vi "WebCAM_Init.vi"(8 "error in (no error)":errorcluster, 10 "PictureBox 2":refnum<k24>(container) caption="PictureBox ------", 11 "Window Title":string="Title") -> (0 "error out":errorcluster, 2 "error initialising":bool, 3 "hwnd":u32, 4 "picture boxx Handle":refnum<k24>)   [LabVIEW 2011]
uses:
  System.Windows.Forms
  user32.dll
  avicap32.dll
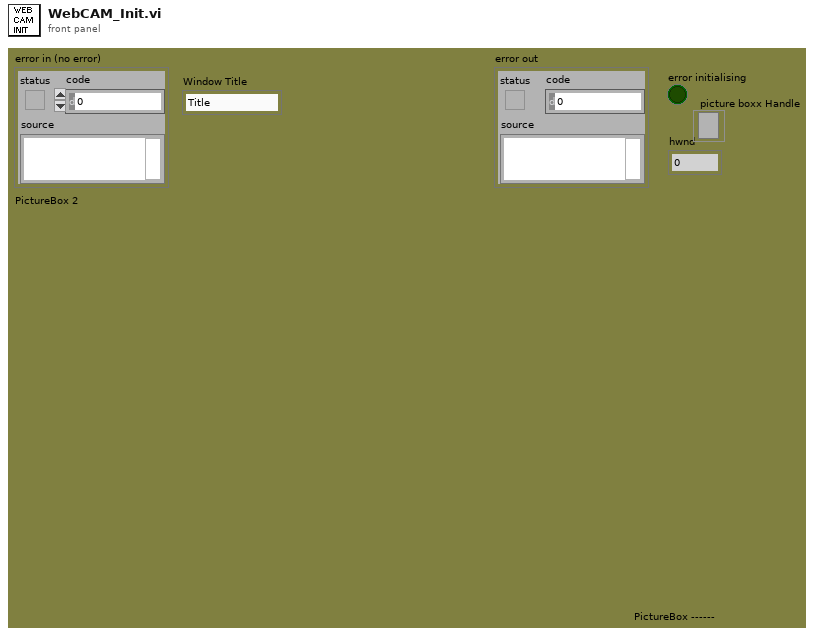
[diagram p1: front panel]
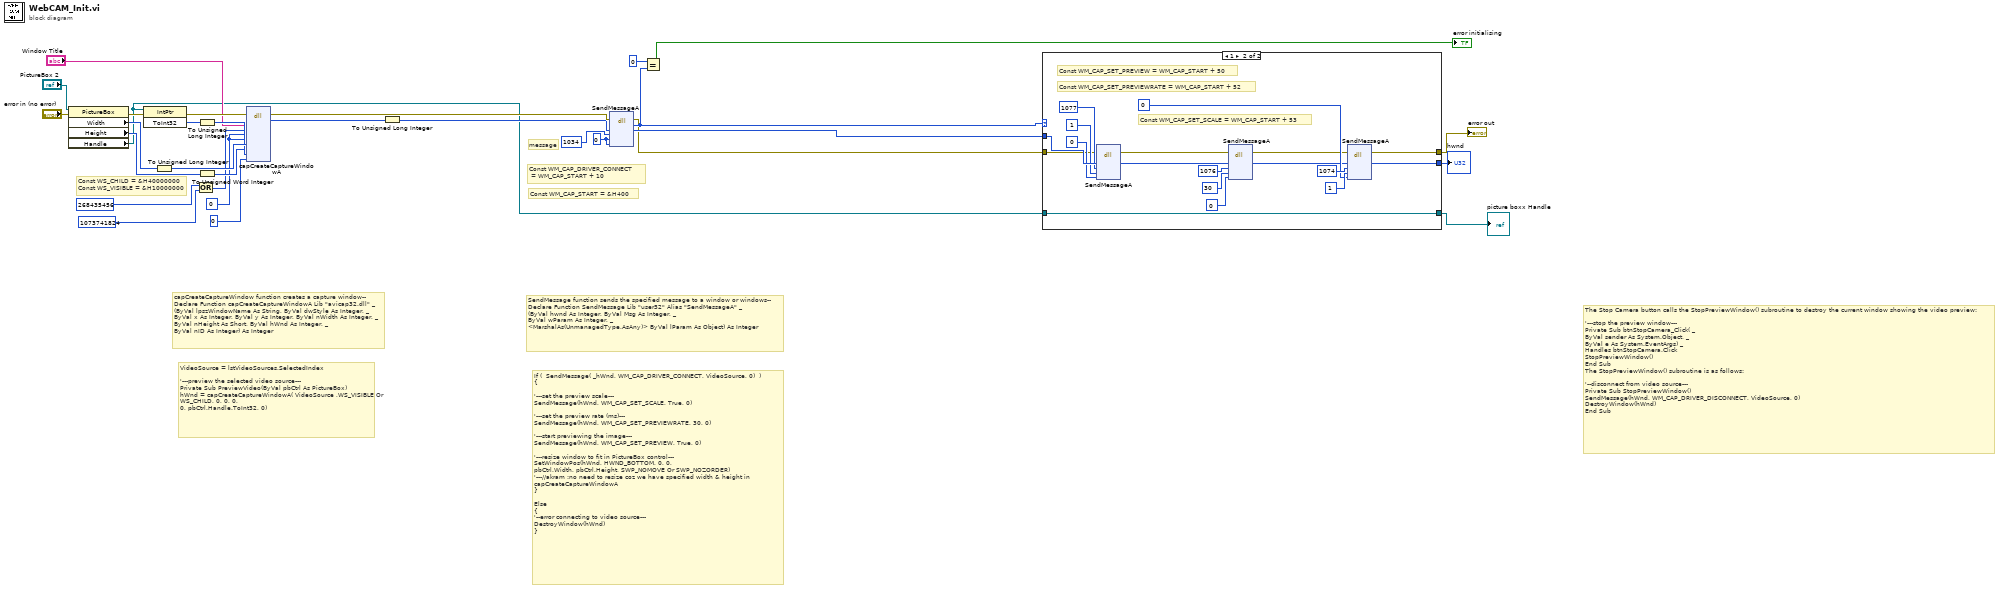
[diagram p0: block diagram]
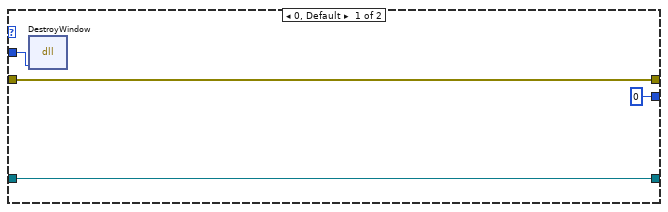
[diagram p2: hidden frame]
diagram:
  w15 = u32 0 ("wParam")
  w18 = u32 0 ("y")
  # "The Stop Camera button calls the StopPreviewWindow() subroutine to destroy the current window showing the video preview:\n\n'---stop the preview window---\nPrivate Sub btnStopCamera_Click( _\nByVal sender As System.Object, _\nByVal e As System.EventArgs) _\nHandles btnStopCamera.Click\nStopPreviewWindow()\nEnd Sub\nThe StopPreviewWindow() subroutine is as follows:\n\n'--disconnect from video source---\nPrivate Sub StopPreviewWindow()\nSendMessage(hWnd, WM_CAP_DRIVER_DISCONNECT, VideoSource, 0)\nDestroyWindow(hWnd)\nEnd Sub"
  # "If (  SendMessage( _hWnd, WM_CAP_DRIVER_CONNECT, VideoSource, 0)  )\n{\n\n'---set the preview scale---\nSendMessage(hWnd, WM_CAP_SET_SCALE, True, 0)\n\n'---set the preview rate (ms)---\nSendMessage(hWnd, WM_CAP_SET_PREVIEWRATE, 30, 0)\n\n'---start previewing the image---\nSendMessage(hWnd, WM_CAP_SET_PREVIEW, True, 0)\n\n'---resize window to fit in PictureBox control---\nSetWindowPos(hWnd, HWND_BOTTOM, 0, 0, \npbCtrl.Width, pbCtrl.Height, SWP_NOMOVE Or SWP_NOZORDER)\n'---//akram :no need to resize coz we have specified width & height in capCreateCaptureWindowA\n}\n\nElse\n{\n'--error connecting to video source---\nDestroyWindow(hWnd)\n}"
  # "Const WM_CAP_START = &H400"
  # "Const WM_CAP_DRIVER_CONNECT\n = WM_CAP_START + 10"
  # "VideoSource = lstVideoSources.SelectedIndex\n\n'---preview the selected video source---\nPrivate Sub PreviewVideo(ByVal pbCtrl As PictureBox)\nhWnd = capCreateCaptureWindowA( VideoSource ,WS_VISIBLE Or WS_CHILD, 0, 0, 0, \n0, pbCtrl.Handle.ToInt32, 0)"
  # "message"
  # "SendMessage function sends the specified message to a window or windows--\nDeclare Function SendMessage Lib \"user32\" Alias \"SendMessageA\" _\n(ByVal hwnd As Integer, ByVal Msg As Integer, _\nByVal wParam As Integer, _\n<MarshalAs(UnmanagedType.AsAny)> ByVal lParam As Object) As Integer"
  # "capCreateCaptureWindow function creates a capture window--\nDeclare Function capCreateCaptureWindowA Lib \"avicap32.dll\" _\n(ByVal lpszWindowName As String, ByVal dwStyle As Integer, _\nByVal x As Integer, ByVal y As Integer, ByVal nWidth As Integer, _\nByVal nHeight As Short, ByVal hWnd As Integer, _\nByVal nID As Integer) As Integer"
  # "Const WS_CHILD = &H40000000\nConst WS_VISIBLE = &H10000000"
  n1 = property class="PictureBox"(reference="PictureBox 2", error in="error in (no error)") -> (error out=w26:errorcluster, "Width"=w27:i32, "Height"=w28:i32, "Handle"=w3:refnum<k24>)  [unwired: 1 out]
  n2 = invoke class="IntPtr" method="ToInt32"(reference=w3, error in=w26) -> (error out=w29:errorcluster, "ToInt32"=w19:i32)  [unwired: 1 in, 1 out]
  n3 = To Unsigned Long Integer(number=w27) -> (unsigned 32bit integer=w25:u32)
  n4 = Or(x=u32 268435456, y=u32 1073741824) -> (x .or. y?=w22:u32)
  n5 = To Unsigned Long Integer(number=w19) -> (unsigned 32bit integer=w24:u32)
  n6 = To Unsigned Word Integer(number=w28) -> (unsigned 16bit integer=w23:u16)
  n7 = dll-call lib="avicap32.dll" fn="capCreateCaptureWindowA"(error in=w29, "lpszWindowName"="Window Title", "dwStyle"=w22, "x"=w18, "y"=w18, "nWidth"=w25, "nHeight"=w23, "hwnd"=w24, "nID"=u32 0) -> (error out=w11:errorcluster, "return type"=w13:i32)  [unwired: 10 in, 1 out]
  n8 = To Unsigned Long Integer(number=w13) -> (unsigned 32bit integer=w8:u32)
  n9 = dll-call lib="user32.dll" fn="SendMessageA"(error in=w11, "hwnd"=w8, "msg"=u32 1034, "wParam"=w15, "lparam"=w15) -> (error out=w10:errorcluster, "return type"=w14:u32, "hwnd"=w12:u32)  [unwired: 5 in, 1 out]
  n10 = Equal?(x=u32 0, y=w14) -> (x = y?=→"error initialising":bool)
  n11 = case shown="1" w14 {
    tunnel: w12 -> [w33 w52]
    tunnel: w10 -> [w34 w38]
    tunnel: [w34 w35] -> w30
    tunnel: w3 -> [w32 w37]
    tunnel: [w32 w37] -> w2
    tunnel: [u32 0 ("hwnd") w36] -> w1
    frame 0, Default {
      n12 = dll-call lib="user32.dll" fn="DestroyWindow"("hwnd"=w33) -> ()  [unwired: 5 in, 2 out]
    }
    frame 1 {
      # "Const WM_CAP_SET_PREVIEW = WM_CAP_START + 50"
      # "Const WM_CAP_SET_PREVIEWRATE = WM_CAP_START + 52"
      # "Const WM_CAP_SET_SCALE = WM_CAP_START + 53"
      n13 = dll-call lib="user32.dll" fn="SendMessageA"(error in=w38, "hwnd"=w52, "msg"=u32 1077, "wParam"=u32 1 ("msg"), "lparam"=u32 0 ("msg")) -> (error out=w45:errorcluster, "hwnd"=w44:u32)  [unwired: 6 in, 1 out]
      n14 = dll-call lib="user32.dll" fn="SendMessageA"(error in=w45, "hwnd"=w44, "msg"=u32 1076, "wParam"=u32 30 ("msg"), "lparam"=u32 0 ("msg")) -> (error out=w40:errorcluster, "hwnd"=w39:u32)  [unwired: 6 in, 1 out]
      n15 = dll-call lib="user32.dll" fn="SendMessageA"(error in=w40, "hwnd"=w39, "msg"=u32 1074, "wParam"=u32 1 ("msg"), "lparam"=u32 0 ("msg")) -> (error out=w35:errorcluster, "hwnd"=w36:u32)  [unwired: 6 in, 1 out]
    }
  }
  "error out" <- w30
  "hwnd" <- w1
  "picture boxx Handle" <- w2
